vi "Check Next Trigger State (non-indexed).vi"(8 "error in (no error)":errorcluster, 10 "States LUT (name -> boolean state)":variant, 11 "TriggerAction in":refnum<class "TriggerAction Q.lvclass">) -> (0 "error out":errorcluster, 2 "Trigger State":bool, 3 "TriggerAction out":refnum<class "TriggerAction Q.lvclass">)   [LabVIEW 2016, in "TriggerAction Q.lvclass"]
uses:
  <userlib>/Common Components/TriggerAction Q/TriggerAction Q/TriggerAction Q.lvclass
  <userlib>/Common Components/TriggerAction Q/TriggerAction Q/TriggerAction Q.lvclass/TriggerAction Q.ctl
  <vilib>/Utility/error.llb/Error Cluster From Error Code.vi
  <vilib>/ErrorRing/Error Ring.xnode
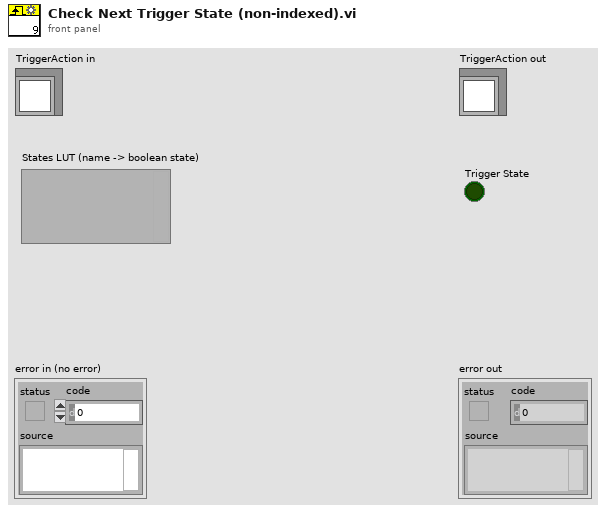
[diagram p1: front panel]
types:
  T1 = typedef "TriggerAction.lvclass/Element Data.ctl" = cluster{"Triggers":cluster{"Triggers for Array AND":string[]}[], "Actions":cluster{"Action Name":string, "Action Data":string}[]}
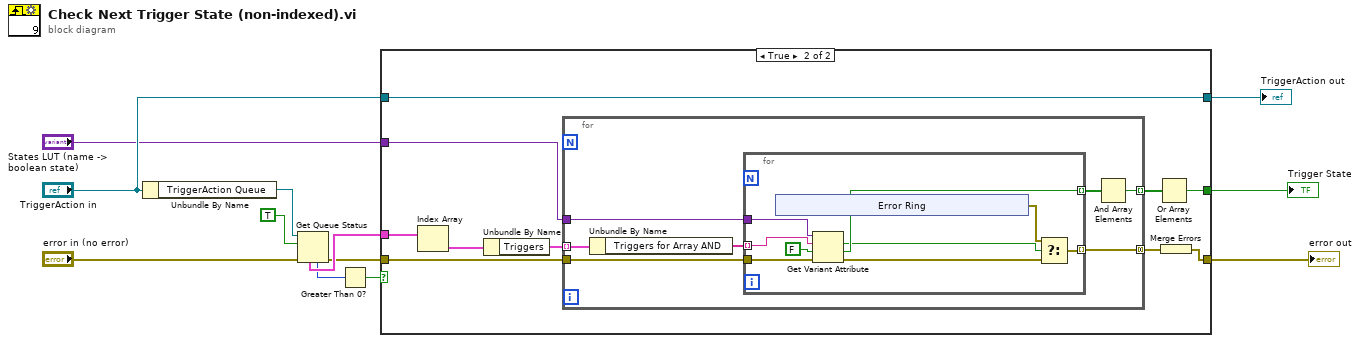
[diagram p0: block diagram]
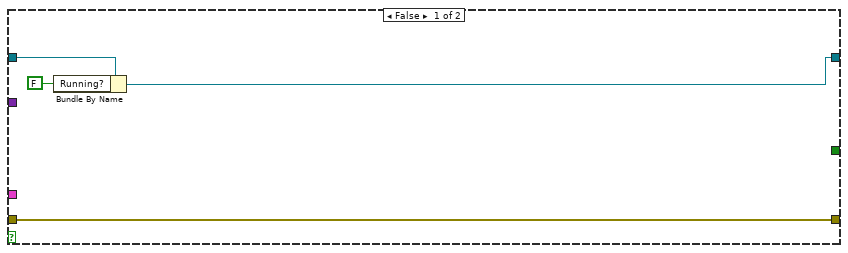
[diagram p2: hidden frame]
diagram:
  n1 = Unbundle By Name("TriggerAction in") -> ("TriggerAction Queue"=w12:refnum<queue>)
  n2 = Get Queue Status(queue=w12, return elements? (F)=TRUE, error in (no error)="error in (no error)") -> (error out=w2:errorcluster, # elements in queue=w8:i32, elements=w10:T1[])  [unwired: 5 out]
  n3 = Greater Than 0?(x=w8) -> (x > 0?=w7:bool)
  n4 = case shown="True" w7 {
    tunnel: w10 -> [_ w26]
    tunnel: "States LUT (name -> boolean state)" -> [_ w23]
    tunnel: [_ w21] -> w9
    tunnel: "TriggerAction in" -> [w16 w20]
    tunnel: [w14 w20] -> w5
    tunnel: w2 -> [w13 w19]
    tunnel: [w13 w17] -> w1
    frame False {
      n5 = Bundle By Name(cluster=w16, "Running?"=FALSE) -> (w14:refnum<class "TriggerAction Q.lvclass">)
    }
    frame True {
      n6 = Index Array(array=w26) -> (element=w25:T1)  [unwired: 1 in]
      n7 = Unbundle By Name(w25) -> ("Triggers"=w24:cluster{"Triggers for Array AND":string[]}[])
      n8 = for {
        tunnel: w24 -> [w32] mode=indexing
        tunnel: w23 -> [w33]
        tunnel: [w29] -> w22 mode=indexing
        tunnel: w19 -> [w28]
        tunnel: [w27] -> w18 mode=concatenating
        n9 = Unbundle By Name(w32) -> ("Triggers for Array AND"=w30:string[])
        n10 = for {
          tunnel: w33 -> [w42]
          tunnel: [w39] -> w31 mode=indexing
          tunnel: w30 -> [w41] mode=indexing
          tunnel: w28 -> [w38]
          tunnel: [w34] -> w27 mode=indexing
          n11 = xnode "Error Ring"() -> ("error out"=w36:errorcluster)
          n12 = Get Variant Attribute(Variant=w42, name=w41, default value (empty Variant)=FALSE, error in=w38) -> (found=w37:bool, value=w39:bool, error out=w35:errorcluster)  [unwired: 1 out]
          n13 = Select(t=w36, s=w37, f=w35) -> (s? t:f=w34:errorcluster)
        }
        n14 = And Array Elements(Boolean array=w31) -> (logical AND=w29:bool)
      }
      n15 = Or Array Elements(Boolean array=w22) -> (logical OR=w21:bool)
      n16 = Merge Errors(w18) -> (w17:errorcluster)
    }
  }
  "error out" <- w1
  "TriggerAction out" <- w5
  "Trigger State" <- w9
